vi "obj_LuaVIEW Task State Instantiator.vi"(0 "method":T1) -> (4 "set for retrieval?":bool, 8 "state object ref":T2, 15 "instantiation error":errorcluster)   [LabVIEW 2012]
doc: "Instantiates a new task state and caches it for retrieval by an asynchronous context. When the latched boolean is reset by retrieval, \"Do Task\", \"Run Task\", and \"Swap Task\" can stop worrying about the task preparations since the task state machine is guaranteed to progress to emptying the preparations object."
uses:
  typedefs/t_LuaVIEW Task State Instantiator Methods.ctl
  typedefs/t_LuaVIEW Task State Pane.ctl
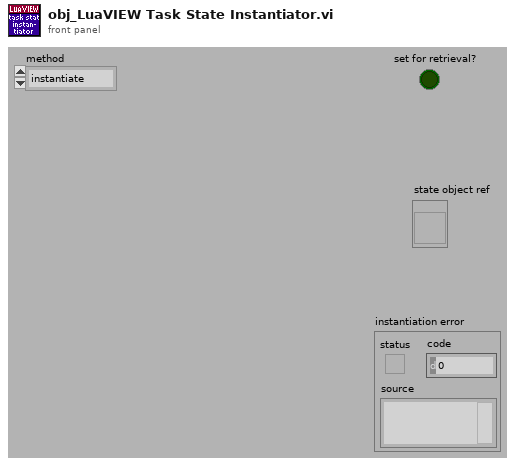
[diagram p1: front panel]
types:
  T1 = typedef "t_LuaVIEW Task State Instantiator Methods.ctl" = enum16{"instantiate", "isset", "retrieve"}
  T2 = typedef "t_LuaVIEW Task State Pane.ctl" = refnum<vi>
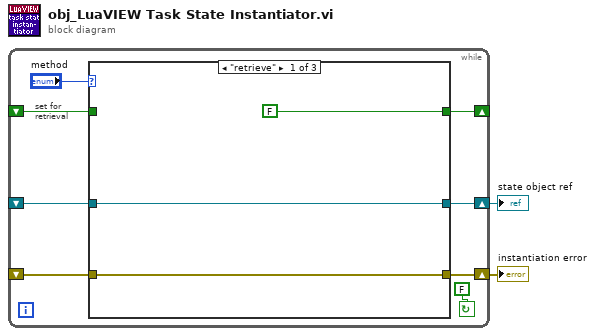
[diagram p0: block diagram]
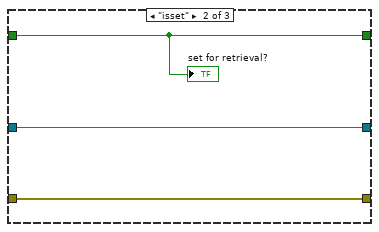
[diagram p2: hidden frame]
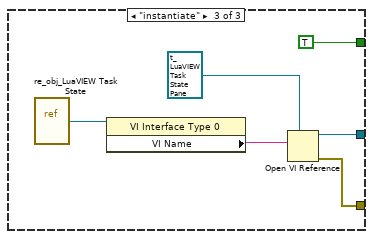
[diagram p3: hidden frame]
diagram:
  n1 = while {
    shift-right: [w8] -> w1
    shift-left: _ -> [w7]
    shift-right: [w4] -> _
    shift-left: _ -> [w3]
    shift-right: [w5] -> w2
    shift-left: _ -> [w6]
    stop <- FALSE continue-if-true
    # "set for\nretrieval"
    n2 = case shown="\"retrieve\"" "method" {
      tunnel: [w13 w16 w20] -> w5
      tunnel: [w12 w15 w22] -> w8
      tunnel: w7 -> [w12 w15 _]
      tunnel: w6 -> [w13 w16 _]
      tunnel: [FALSE w14 TRUE] -> w4
      tunnel: w3 -> [_ w14 _]
      frame "retrieve" {
      }
      frame "isset" {
        "set for retrieval?" <- w14
      }
      frame "instantiate" {
        n3 = vi-ref "re_obj_LuaVIEW Task State.vi"() -> ("vi reference"=w18:refnum<vi>)
        n4 = property class="VI Interface Type 0"(reference=w18) -> ("VI Name"=w17:string)  [unwired: 1 in, 2 out]
        n5 = Open VI Reference(type specifier VI Refnum (for type only)=T2 refnum ("state object pane"), vi path=w17) -> (vi reference=w22:T2, error out=w20:errorcluster)  [unwired: 4 in]
      }
    }
  }
  "instantiation error" <- w2
  "state object ref" <- w1
